vi "Build Status.vi"(8 "error in (no error)":errorcluster, 11 "Sequencing in":refnum<class "Sequencing.lvclass">) -> (0 "error out":errorcluster, 2 "Sequencing Status":T1 {"Sequences"."CRC32" format="%08x"}, 3 "Sequencing out":refnum<class "Sequencing.lvclass">)   [LabVIEW 2020, in "VolatusSeq.lvlib" / "Sequencing.lvclass"]
uses:
  Sequencing.lvclass
  Sequencing Status.ctl
  Sequence Status Extended.ctl
  Sequence Status.ctl
  Sequence Time.ctl
  Sequencing.lvclass/Sequencing.ctl
  Sequence/Sequence.lvclass/Sequence.ctl
  VolatusSeq.lvlib
  Sequence/Sequence.lvclass
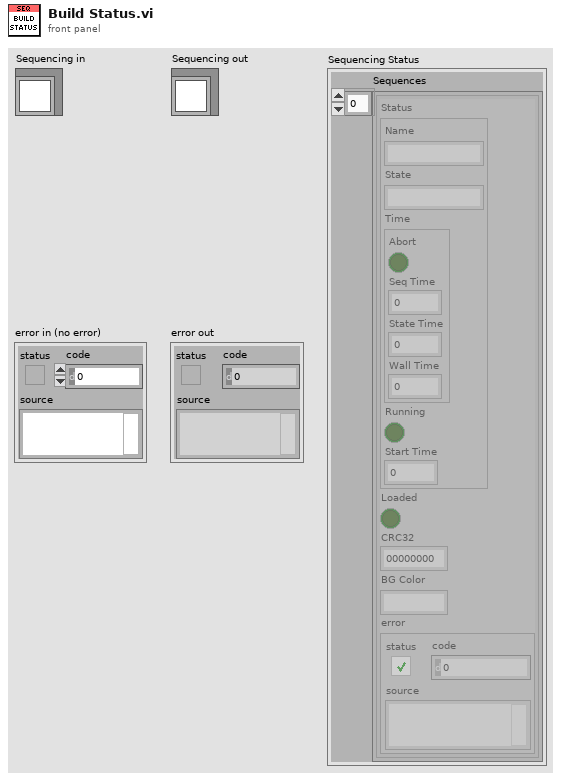
[diagram p1: front panel]
types:
  T1 = typedef "VolatusSeq.lvlib/Sequencing Status.ctl" = cluster{"Sequences":T2[]}
  T2 = typedef "VolatusSeq.lvlib/Sequence Status Extended.ctl" = cluster{"Status":T3, "Loaded":bool, "CRC32":u32, "BG Color":string, "error":errorcluster}
  T3 = typedef "VolatusSeq.lvlib/Sequence Status.ctl" = cluster{"Name":string, "State":string, "Time":T4, "Running":bool, "Start Time":dbl}
  T4 = typedef "VolatusSeq.lvlib/Sequence Time.ctl" = cluster{"Abort":bool, "Seq Time":dbl, "State Time":dbl, "Wall Time":dbl}
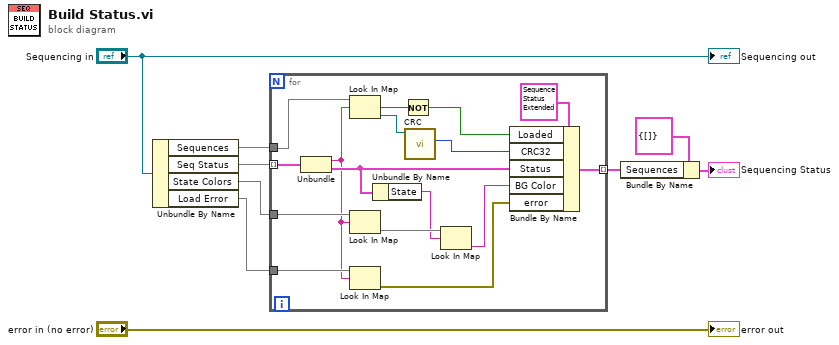
[diagram p0: block diagram]
diagram:
  n1 = Unbundle By Name("Sequencing in") -> ("Sequences"=w4:map{string, refnum<class "Sequence.lvclass">}, "Seq Status"=w5:map{string, T3}, "State Colors"=w2:map{string, map{string, string}}, "Load Error"=w1:map{string, errorcluster})
  n2 = for {
    tunnel: w5 -> [w25] mode=indexing
    tunnel: w4 -> [w24]
    tunnel: [w21] -> w3 mode=indexing
    tunnel: w2 -> [w20]
    tunnel: w1 -> [w12]
    n3 = Unbundle(w25) -> ("Name"=w11:string, "Status"=w18:T3)
    n4 = Look In Map(map=w24, key=w11) -> (key not found?=w23:bool, value=w14:refnum<class "Sequence.lvclass">)  [unwired: 1 in]
    n5 = Look In Map(map=w20, key=w11) -> (value=w19:map{string, string})  [unwired: 1 in, 1 out]
    n6 = Look In Map(map=w12, key=w11) -> (value=w10:errorcluster)  [unwired: 1 in, 1 out]
    n7 = Unbundle By Name(w18) -> ("State"=w17:string)
    n8 = Not(x=w23) -> (.not. x?=w15:bool)
    n9 = call "CRC.vi"("Sequence in"=w14) -> ("CRC"=w13:u32)  [unwired: 8 in, 2 out]
    n10 = Look In Map(map=w19, key=w17) -> (value=w16:string)  [unwired: 1 in, 1 out]
    n11 = Bundle By Name(cluster=T2 {"Status"={"Name"="", "State"="", "Time"={"Abort"=FALSE, "Seq Time"=0.0, "State Time"=0.0, "Wall Time"=0.0}, "Running"=FALSE, "Start Time"=0.0}, "Loaded"=FALSE, "CRC32"=0, "BG Color"="", "error"={"status"=FALSE, "code"=0, "source"=""}} ("Sequence Status Extended"), "Loaded"=w15, "CRC32"=w13, "Status"=w18, "BG Color"=w16, "error"=w10) -> (w21:T2)
  }
  n12 = Bundle By Name(cluster=T1 {"Sequences"=[]} ("Sequencing Status"), "Sequences"=w3) -> (→"Sequencing Status":T1)
  "error out" <- "error in (no error)"
  "Sequencing out" <- "Sequencing in"
